vi "Global-Gserver-Instance.vi"() -> ()   [LabVIEW 2020, in "Sgraph_lib_V1.lvlib" / "Gserver.lvclass"]
uses:
  Gserver.lvclass
panel:
  out "Gserver instance":refnum<data-value>
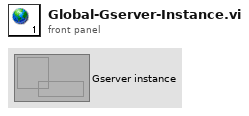
[diagram p1: front panel]
diagram:
